vi "Quiz.vi"() -> ()   [LabVIEW 2020]
uses:
  <vilib>/Utility/error.llb/whitespace.ctl
panel:
  in  "array 3":string[](array[string])
  in  "array 2":string[](array[string])
  in  "array":string[](array[string])
  out "x+y":i16
  in  "Boolean 6":bool
  in  "Boolean 5":bool
  in  "Boolean 4":bool
  out "Boolean 3":bool
  out "Boolean 2":bool
  out "Boolean":bool
  out "Array 2":string[](array[string])
  out "number":dbl
  out "Numeric":i32
  in  "?":string
  in  "?":bool
  out "?":string
  in  "?":string
  # "Ingresar trama"
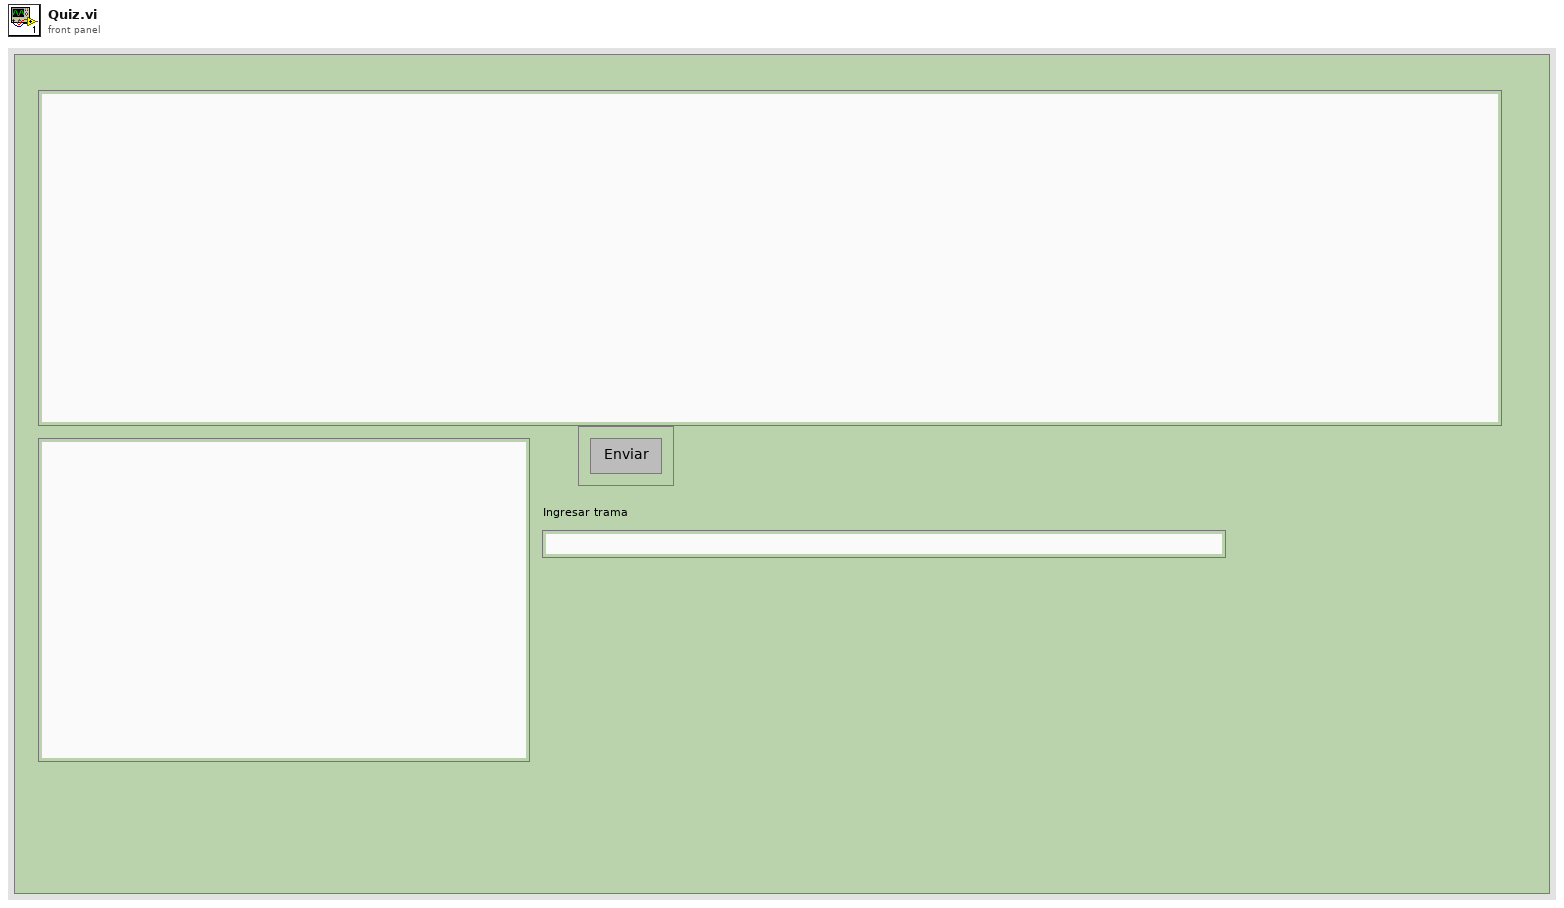
[diagram p1: front panel]
types:
  T1 = enum8{"Enabled", "Disabled", "Disabled and Grayed Out"}
  T2 = typedef "whitespace.ctl" = u16
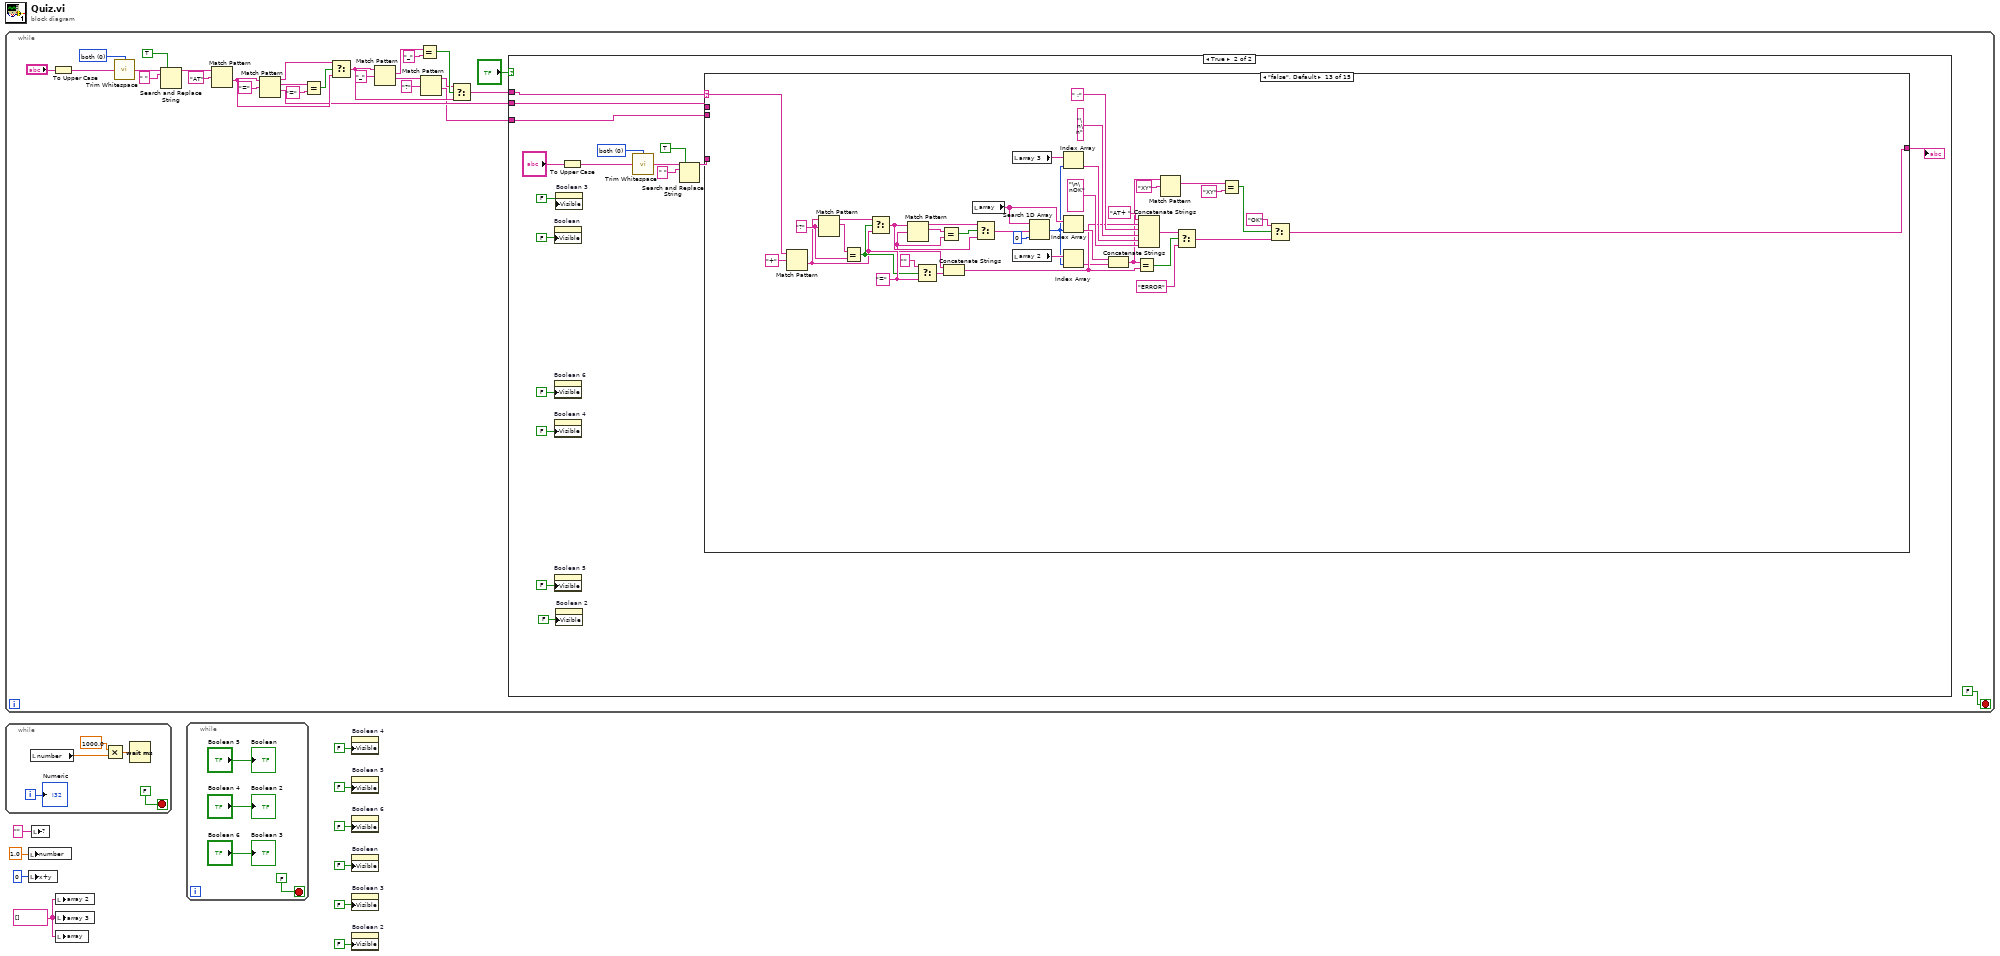
[diagram p0: block diagram]
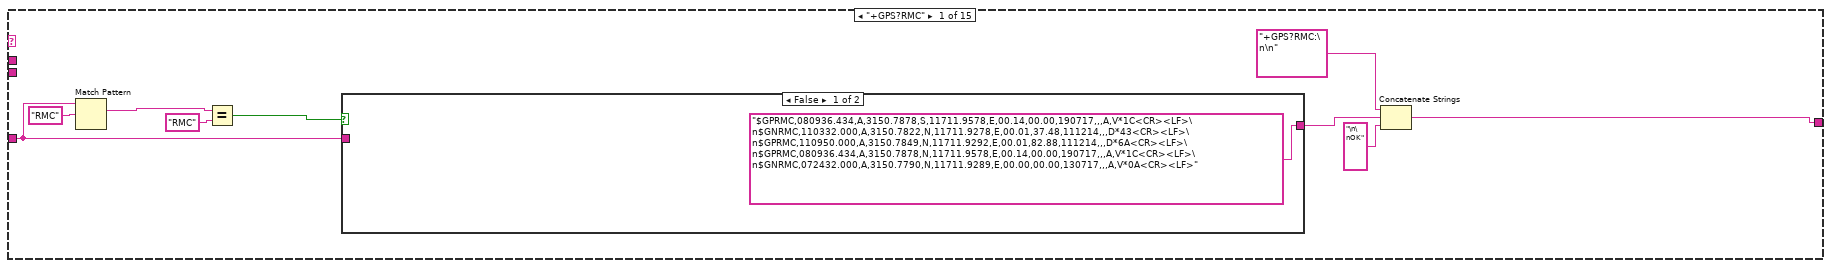
[diagram p3: hidden frame]
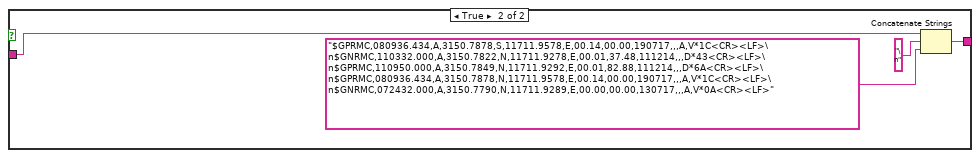
[diagram p4: hidden frame]
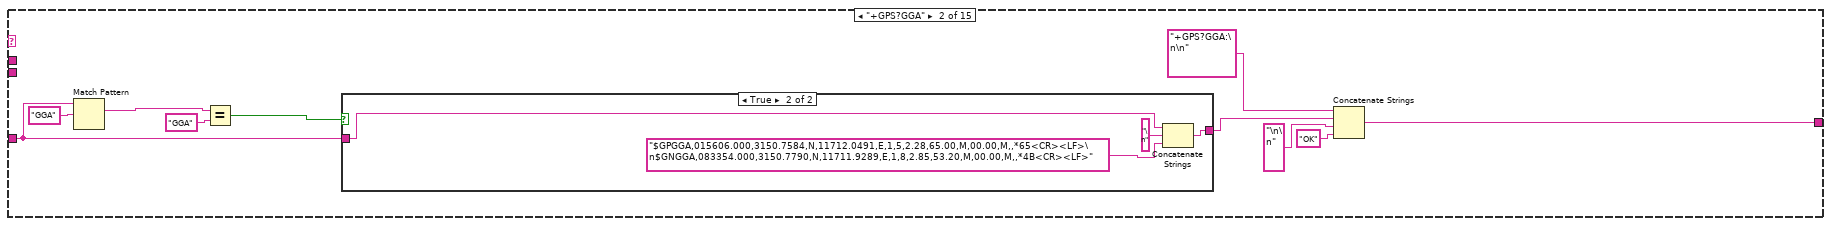
[diagram p5: hidden frame]
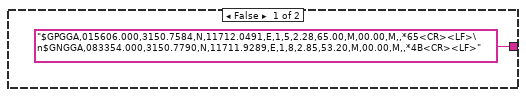
[diagram p6: hidden frame]
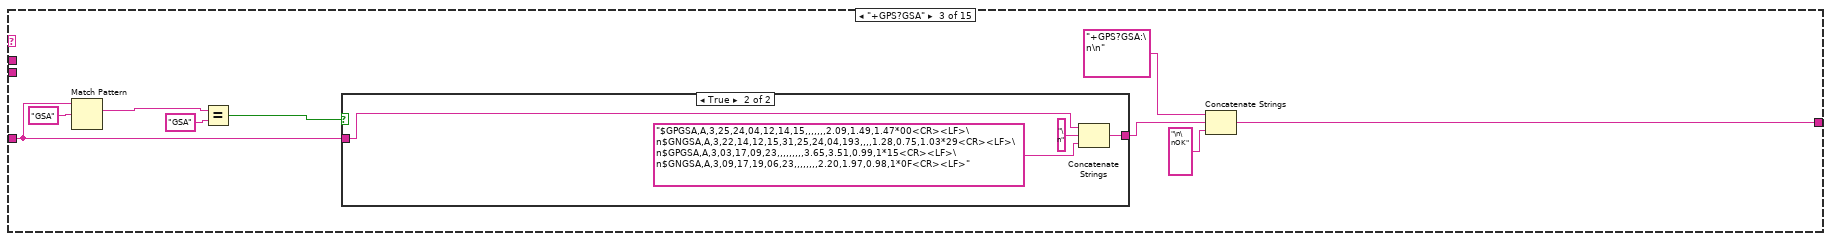
[diagram p7: hidden frame]
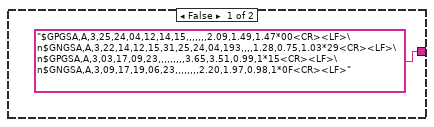
[diagram p8: hidden frame]
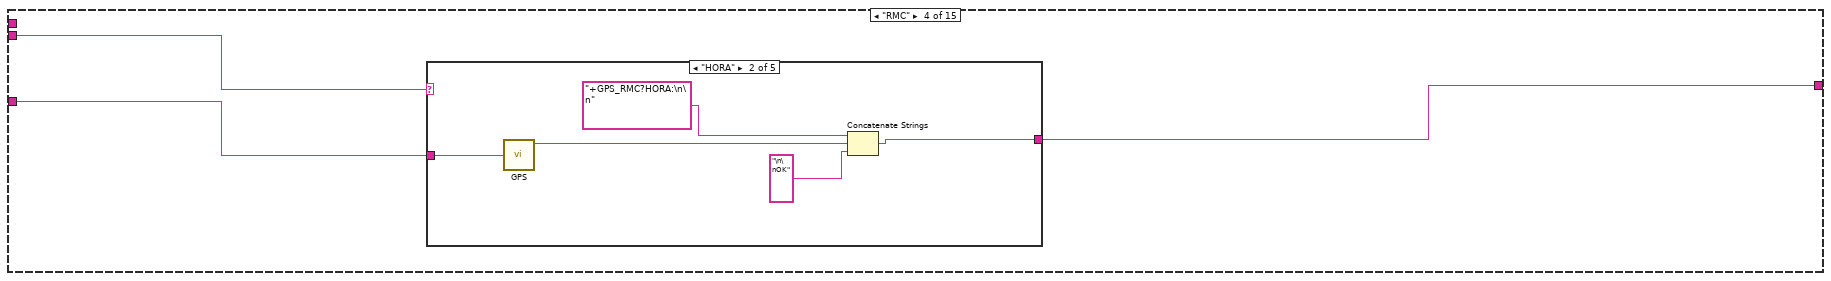
[diagram p9: hidden frame]
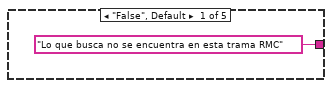
[diagram p10: hidden frame]
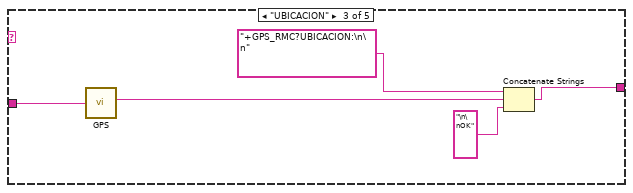
[diagram p11: hidden frame]
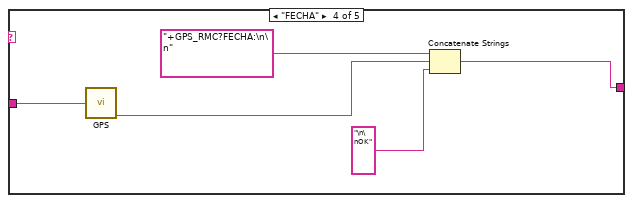
[diagram p12: hidden frame]
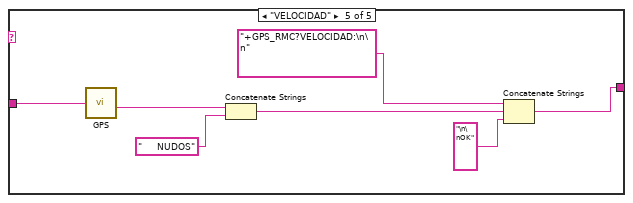
[diagram p13: hidden frame]
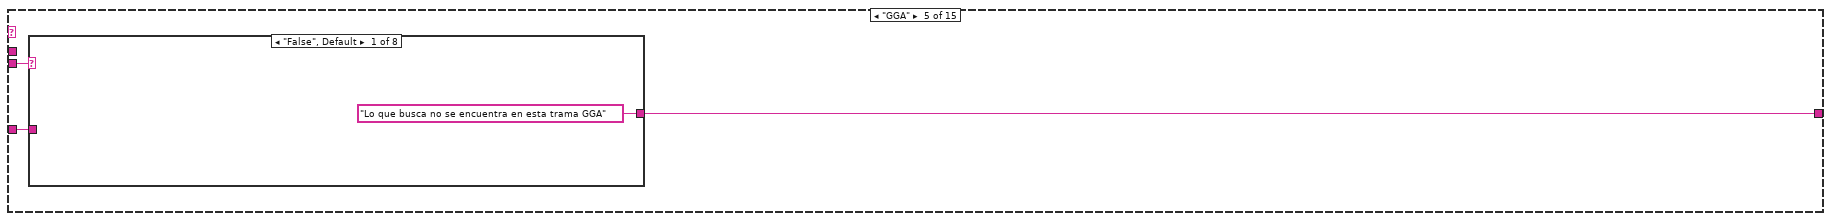
[diagram p14: hidden frame]
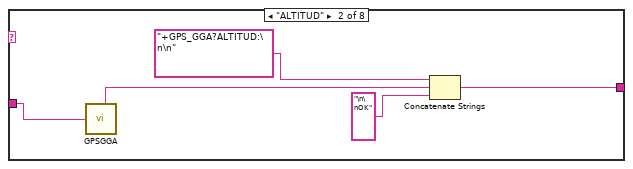
[diagram p15: hidden frame]
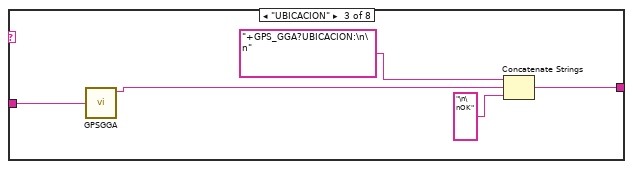
[diagram p16: hidden frame]
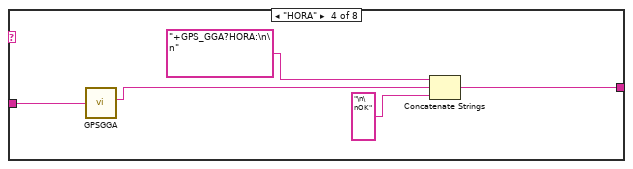
[diagram p17: hidden frame]
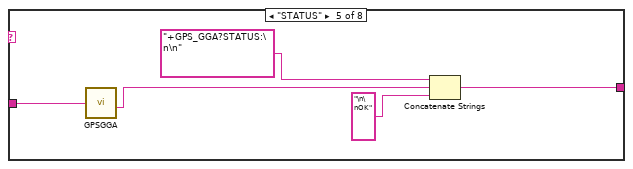
[diagram p18: hidden frame]
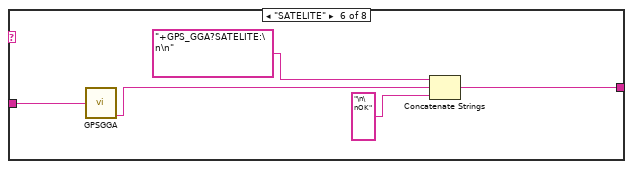
[diagram p19: hidden frame]
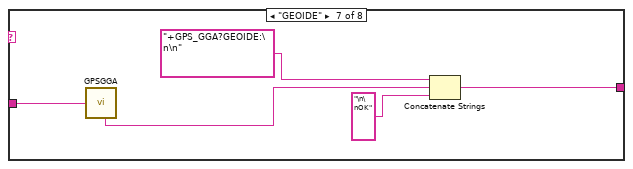
[diagram p20: hidden frame]
diagram:
  w1 = string[] [] ("Array")
  n1 = while {
    stop <- FALSE stop-if-true
    w17 = T2 0 items=["both", "start of string", "end of string"] ("location (both)")
    n2 = To Upper Case(1:"?") -> (0:w13:string)
    n3 = call <vilib>:"Trim Whitespace.vi"("string"=w13, "location (both)"=w17) -> ("trimmed string"=w16:string)
    n4 = Search and Replace String(replace all?=TRUE ("replace all? (F)"), input string=w16, search string=" ") -> (result string=w12:string)  [unwired: 5 in, 3 out]
    n5 = Match Pattern(string=w12, regular expression="AT" ("string")) -> (after substring=w28:string)  [unwired: 1 in, 3 out]
    n6 = Match Pattern(string=w28, regular expression="=") -> (before substring=w29:string, match substring=w32:string, after substring=w27:string)  [unwired: 1 in, 1 out]
    n7 = Equal?(x=w32, y="=") -> (x = y?=w30:bool)
    n8 = Select(t=w29, s=w30, f=w28) -> (s? t:f=w22:string)
    n9 = Match Pattern(string=w22, regular expression="_") -> (match substring=w25:string, after substring=w21:string)  [unwired: 1 in, 2 out]
    n10 = Equal?(x=w25, y="_") -> (x = y?=w23:bool)
    n11 = Match Pattern(string=w21, regular expression="?") -> (before substring=w19:string, after substring=w18:string)  [unwired: 1 in, 2 out]
    n12 = Select(t=w19, s=w23, f=w22) -> (s? t:f=w11:string)
    n13 = case shown="True" "?" {
      tunnel: w11 -> [_ w54]
      tunnel: w27 -> [_ w53]
      tunnel: w18 -> [_ w51]
      frame False {
      }
      frame True {
        w46 = T2 0 items=["both", "start of string", "end of string"] ("location (both)")
        n14 = property on="Boolean" class="Bool (strict)"("Visible"=FALSE) -> ()  [unwired: 2 in, 2 out]
        n15 = property on="Boolean 6" class="Bool (strict)"("Visible"=FALSE) -> ()  [unwired: 2 in, 2 out]
        n16 = property on="Boolean 4" class="Bool (strict)"("Visible"=FALSE) -> ()  [unwired: 2 in, 2 out]
        n17 = property on="Boolean 5" class="Bool (strict)"("Visible"=FALSE) -> ()  [unwired: 2 in, 2 out]
        n18 = property on="Boolean 3" class="Bool (strict)"("Visible"=FALSE) -> ()  [unwired: 2 in, 2 out]
        n19 = property on="Boolean 2" class="Bool (strict)"("Visible"=FALSE) -> ()  [unwired: 2 in, 2 out]
        n20 = To Upper Case(1:"?") -> (0:w50:string)
        n21 = call <vilib>:"Trim Whitespace.vi"("string"=w50, "location (both)"=w46) -> ("trimmed string"=w47:string)
        n22 = Search and Replace String(replace all?=TRUE ("replace all? (F)"), input string=w47, search string=" ") -> (result string=w45:string)  [unwired: 5 in, 3 out]
        n23 = case shown="\"false\", Default" w54 {
          selector: w54 -> [_ _ _ _ _ _ _ _ _ _ _ _ w378 _ _]
          tunnel: [w56 w71 w85 w98 w124 w164 w255 w262 w274 "" "" w318 w340 w379 "AT:\n\nOk"] -> w52
          tunnel: w45 -> [w61 w74 w88 w100 w126 w162 _ _ _ _ _ _ _ _ _]
          tunnel: w53 -> [_ _ _ _ _ _ _ w268 _ _ _ w316 _ _ _]
          tunnel: w51 -> [_ _ _ w99 w125 w165 _ _ _ _ _ _ _ _ _]
          frame "+GPS?RMC" {
            n24 = Match Pattern(string=w61, regular expression="RMC") -> (match substring=w59:string)  [unwired: 1 in, 3 out]
            n25 = Equal?(x=w59, y="RMC") -> (x = y?=w62:bool)
            n26 = case shown="False" w62 {
              tunnel: w61 -> [_ w66]
              tunnel: ["$GPRMC,080936.434,A,3150.7878,S,11711.9578,E,00.14,00.00,190717,,,A,V*1C<CR><LF>\n$GNRMC,110332.000,A,3150.7822,N,11711.9278,E,00.01,37.48,111214,,,D*43<CR><LF>\n$GPRMC,110950.000,A,3150.7849,N,11711.9292,E,00.01,82.88,111214,,,D*6A<CR><LF>\n$GPRMC,080936.434,A,3150.7878,N,11711.9578,E,00.14,00.00,190717,,,A,V*1C<CR><LF>\n$GNRMC,072432.000,A,3150.7790,N,11711.9289,E,00.00,00.00,130717,,,A,V*0A<CR><LF>" w68] -> w57
              frame False {
              }
              frame True {
                n27 = Concatenate Strings(w66, "\n" ("string"), "$GPRMC,080936.434,A,3150.7878,S,11711.9578,E,00.14,00.00,190717,,,A,V*1C<CR><LF>\n$GNRMC,110332.000,A,3150.7822,N,11711.9278,E,00.01,37.48,111214,,,D*43<CR><LF>\n$GPRMC,110950.000,A,3150.7849,N,11711.9292,E,00.01,82.88,111214,,,D*6A<CR><LF>\n$GPRMC,080936.434,A,3150.7878,N,11711.9578,E,00.14,00.00,190717,,,A,V*1C<CR><LF>\n$GNRMC,072432.000,A,3150.7790,N,11711.9289,E,00.00,00.00,130717,,,A,V*0A<CR><LF>") -> (w68:string)
              }
            }
            n28 = Concatenate Strings("+GPS?RMC:\n\n" ("string"), w57, "\n\nOK" ("string")) -> (w56:string)
          }
          frame "+GPS?GGA" {
            n29 = Match Pattern(string=w74, regular expression="GGA") -> (match substring=w75:string)  [unwired: 1 in, 3 out]
            n30 = Equal?(x=w75, y="GGA") -> (x = y?=w76:bool)
            n31 = case shown="True" w76 {
              tunnel: w74 -> [_ w81]
              tunnel: ["$GPGGA,015606.000,3150.7584,N,11712.0491,E,1,5,2.28,65.00,M,00.00,M,,*65<CR><LF>\n$GNGGA,083354.000,3150.7790,N,11711.9289,E,1,8,2.85,53.20,M,00.00,M,,*4B<CR><LF>" w83] -> w72
              frame False {
              }
              frame True {
                n32 = Concatenate Strings(w81, "\n" ("string"), "$GPGGA,015606.000,3150.7584,N,11712.0491,E,1,5,2.28,65.00,M,00.00,M,,*65<CR><LF>\n$GNGGA,083354.000,3150.7790,N,11711.9289,E,1,8,2.85,53.20,M,00.00,M,,*4B<CR><LF>") -> (w83:string)
              }
            }
            n33 = Concatenate Strings("+GPS?GGA:\n\n" ("string"), w72, "\n\n" ("string"), "OK" ("string")) -> (w71:string)
          }
          frame "+GPS?GSA" {
            n34 = Match Pattern(string=w88, regular expression="GSA") -> (match substring=w89:string)  [unwired: 1 in, 3 out]
            n35 = Equal?(x=w89, y="GSA") -> (x = y?=w90:bool)
            n36 = case shown="True" w90 {
              tunnel: w88 -> [_ w95]
              tunnel: ["$GPGSA,A,3,25,24,04,12,14,15,,,,,,,2.09,1.49,1.47*00<CR><LF>\n$GNGSA,A,3,22,14,12,15,31,25,24,04,193,,,,1.28,0.75,1.03*29<CR><LF>\n$GPGSA,A,3,03,17,09,23,,,,,,,,,3.65,3.51,0.99,1*15<CR><LF>\n$GNGSA,A,3,09,17,19,06,23,,,,,,,,2.20,1.97,0.98,1*0F<CR><LF>" w96] -> w86
              frame False {
              }
              frame True {
                n37 = Concatenate Strings(w95, "\n" ("string"), "$GPGSA,A,3,25,24,04,12,14,15,,,,,,,2.09,1.49,1.47*00<CR><LF>\n$GNGSA,A,3,22,14,12,15,31,25,24,04,193,,,,1.28,0.75,1.03*29<CR><LF>\n$GPGSA,A,3,03,17,09,23,,,,,,,,,3.65,3.51,0.99,1*15<CR><LF>\n$GNGSA,A,3,09,17,19,06,23,,,,,,,,2.20,1.97,0.98,1*0F<CR><LF>") -> (w96:string)
              }
            }
            n38 = Concatenate Strings("+GPS?GSA:\n\n" ("string"), w86, "\n\nOK" ("string")) -> (w85:string)
          }
          frame "RMC" {
            n39 = case shown="\"HORA\"" w99 {
              tunnel: w100 -> [_ w106 w111 w116 w123]
              tunnel: ["Lo que busca no se encuentra en esta trama RMC" w102 w107 w112 w117] -> w98
              frame "False", Default {
              }
              frame "HORA" {
                n40 = call "GPS.vi"("String"=w106) -> ("Hora"=w103:string)  [unwired: 3 out]
                n41 = Concatenate Strings("+GPS_RMC?HORA:\n\n" ("string"), w103, "\n\nOK" ("string")) -> (w102:string)
              }
              frame "UBICACION" {
                n42 = call "GPS.vi"("String"=w111) -> ("Ubicación"=w108:string)  [unwired: 3 out]
                n43 = Concatenate Strings("+GPS_RMC?UBICACION:\n\n" ("string"), w108, "\n\nOK" ("string")) -> (w107:string)
              }
              frame "FECHA" {
                n44 = call "GPS.vi"("String"=w116) -> ("Fecha"=w113:string)  [unwired: 3 out]
                n45 = Concatenate Strings("+GPS_RMC?FECHA:\n\n" ("string"), w113, "\n\nOK" ("string")) -> (w112:string)
              }
              frame "VELOCIDAD" {
                n46 = call "GPS.vi"("String"=w123) -> ("Velocidad"=w121:string)  [unwired: 3 out]
                n47 = Concatenate Strings(w121, "     NUDOS" ("string")) -> (w118:string)
                n48 = Concatenate Strings("+GPS_RMC?VELOCIDAD:\n\n" ("string"), w118, "\n\nOK" ("string")) -> (w117:string)
              }
            }
          }
          frame "GGA" {
            n49 = case shown="\"False\", Default" w125 {
              tunnel: w126 -> [_ w132 w137 w142 w147 w152 w157 _]
              tunnel: ["Lo que busca no se encuentra en esta trama GGA" w129 w133 w138 w143 w148 w154 w158] -> w124
              frame "False", Default {
              }
              frame "ALTITUD" {
                n50 = call "GPSGGA.vi"("String"=w132) -> ("Altitud"=w128:string)  [unwired: 5 out]
                n51 = Concatenate Strings("+GPS_GGA?ALTITUD:\n\n" ("string"), w128, "\n\nOK" ("string")) -> (w129:string)
              }
              frame "UBICACION" {
                n52 = call "GPSGGA.vi"("String"=w137) -> ("Ubicación"=w134:string)  [unwired: 5 out]
                n53 = Concatenate Strings("+GPS_GGA?UBICACION:\n\n" ("string"), w134, "\n\nOK" ("string")) -> (w133:string)
              }
              frame "HORA" {
                n54 = call "GPSGGA.vi"("String"=w142) -> ("Hora"=w139:string)  [unwired: 5 out]
                n55 = Concatenate Strings("+GPS_GGA?HORA:\n\n" ("string"), w139, "\n\nOK" ("string")) -> (w138:string)
              }
              frame "STATUS" {
                n56 = call "GPSGGA.vi"("String"=w147) -> ("Fix Status"=w144:string)  [unwired: 5 out]
                n57 = Concatenate Strings("+GPS_GGA?STATUS:\n\n" ("string"), w144, "\n\nOK" ("string")) -> (w143:string)
              }
              frame "SATELITE" {
                n58 = call "GPSGGA.vi"("String"=w152) -> ("# Satelite"=w149:string)  [unwired: 5 out]
                n59 = Concatenate Strings("+GPS_GGA?SATELITE:\n\n" ("string"), w149, "\n\nOK" ("string")) -> (w148:string)
              }
              frame "GEOIDE" {
                n60 = call "GPSGGA.vi"("String"=w157) -> ("Sep Geoide"=w153:string)  [unwired: 5 out]
                n61 = Concatenate Strings("+GPS_GGA?GEOIDE:\n\n" ("string"), w153, "\n\nOK" ("string")) -> (w154:string)
              }
              frame "VELOCIDAD" {
                n62 = Concatenate Strings("+GPS_GGA?VELOCIDAD:\n\n" ("string"), "La trama GGA no tiene velocidad", "\n\nOK" ("string")) -> (w158:string)
              }
            }
          }
          frame "GSA" {
            n63 = call "GPSGSA.vi"("string"=w162) -> ("Array"=→"Array 2":string[])
            n64 = case shown="\"SATELITE1\"" w165 {
              tunnel: ["Lo que busca no se encuentra en la trama GSA" w167 w173 w180 w185 w192 w198 w204 w210 w216 w222 w228 w234 w240 w245 w250] -> w164
              frame "False", Default {
              }
              frame "MODO" {
                n65 = local read "Array 2"() -> (w172:string[])
                n66 = Index Array(array=w172, index=0) -> (element=w168:string)
                n67 = Concatenate Strings("+GPS_GSA?MODO:\n\n" ("string"), w168, "\n\nOK" ("string")) -> (w167:string)
              }
              frame "STATUS" {
                n68 = local read "Array 2"() -> (w178:string[])
                n69 = Index Array(array=w178, index=1) -> (element=w174:string)
                n70 = Concatenate Strings("+GPS_GSA?STATUS:\n\n" ("string"), w174, "\n\nOK" ("string")) -> (w173:string)
              }
              frame "SATELITE1" {
                n71 = local read "Array 2"() -> (w184:string[])
                n72 = Index Array(array=w184, index=2) -> (element=w179:string)
                n73 = Concatenate Strings("+GPS_GSA?SATELITE1:\n\n" ("string"), w179, "\n\nOK" ("string")) -> (w180:string)
              }
              frame "SATELITE2" {
                n74 = local read "Array 2"() -> (w190:string[])
                n75 = Index Array(array=w190, index=3) -> (element=w186:string)
                n76 = Concatenate Strings("+GPS_GSA?SATELITE2:\n\n" ("string"), w186, "\n\nOK" ("string")) -> (w185:string)
              }
              frame "SATELITE3" {
                n77 = local read "Array 2"() -> (w196:string[])
                n78 = Index Array(array=w196, index=4) -> (element=w191:string)
                n79 = Concatenate Strings("+GPS_GSA?SATELITE3:\n\n" ("string"), w191, "\n\nOK" ("string")) -> (w192:string)
              }
              frame "SATELITE4" {
                n80 = local read "Array 2"() -> (w202:string[])
                n81 = Index Array(array=w202, index=5) -> (element=w197:string)
                n82 = Concatenate Strings("+GPS_GSA?SATELITE4:\n\n" ("string"), w197, "\n\nOK" ("string")) -> (w198:string)
              }
              frame "SATELITE5" {
                n83 = local read "Array 2"() -> (w208:string[])
                n84 = Index Array(array=w208, index=6) -> (element=w203:string)
                n85 = Concatenate Strings("+GPS_GSA?SATELITE5:\n\n" ("string"), w203, "\n\nOK" ("string")) -> (w204:string)
              }
              frame "SATELITE6" {
                n86 = local read "Array 2"() -> (w214:string[])
                n87 = Index Array(array=w214, index=7) -> (element=w209:string)
                n88 = Concatenate Strings("+GPS_GSA?SATELITE6:\n\n" ("string"), w209, "\n\nOK" ("string")) -> (w210:string)
              }
              frame "SATELITE7" {
                n89 = local read "Array 2"() -> (w220:string[])
                n90 = Index Array(array=w220, index=8) -> (element=w215:string)
                n91 = Concatenate Strings("+GPS_GSA?SATELITE7:\n\n" ("string"), w215, "\n\nOK" ("string")) -> (w216:string)
              }
              frame "SATELITE8" {
                n92 = local read "Array 2"() -> (w226:string[])
                n93 = Index Array(array=w226, index=9) -> (element=w221:string)
                n94 = Concatenate Strings("+GPS_GSA?SATELITE8:\n\n" ("string"), w221, "\n\nOK" ("string")) -> (w222:string)
              }
              frame "SATELITE9" {
                n95 = local read "Array 2"() -> (w232:string[])
                n96 = Index Array(array=w232, index=10) -> (element=w227:string)
                n97 = Concatenate Strings("+GPS_GSA?SATELITE9:\n\n" ("string"), w227, "\n\nOK" ("string")) -> (w228:string)
              }
              frame "SATELITE10" {
                n98 = local read "Array 2"() -> (w238:string[])
                n99 = Index Array(array=w238, index=11) -> (element=w233:string)
                n100 = Concatenate Strings("+GPS_GSA?SATELITE10:\n\n" ("string"), w233, "\n\nOK" ("string")) -> (w234:string)
              }
              frame "SATELITE11" {
                n101 = local read "Array 2"() -> (w244:string[])
                n102 = Index Array(array=w244, index=12) -> (element=w239:string)
                n103 = Concatenate Strings("+GPS_GSA?SATELITE11:\n\n" ("string"), w239, "\n\nOK" ("string")) -> (w240:string)
              }
              frame "VELOCIDAD" {
                n104 = Concatenate Strings("+GPS_GSA?VELOCIDAD:\n\n" ("string"), "La trama GSA no tiene velocidad", "\n\nOK" ("string")) -> (w245:string)
              }
              frame "SATELITE12" {
                n105 = local read "Array 2"() -> (w254:string[])
                n106 = Index Array(array=w254, index=13) -> (element=w249:string)
                n107 = Concatenate Strings("+GPS_GSA?SATELITE12:\n\n" ("string"), w249, "\n\nOK" ("string")) -> (w250:string)
              }
            }
          }
          frame "+TIMER" {
            n108 = Format Date/Time String() -> (date/time string=w258:string)  [unwired: 3 in]
            n109 = Concatenate Strings(w258, "\n\n" ("string"), "OK" ("string")) -> (w256:string)
            n110 = Concatenate Strings("+TIMER:\n\n" ("string"), w256) -> (w255:string)
          }
          frame "+CONT" {
            n111 = Fract/Exp String To Number(string=w268, default (0 dbl)=1.0 ("default (0 DBL)")) -> (number=w265:dbl)  [unwired: 2 in, 1 out]
            "number" <- w265
            n112 = Number To Decimal String(number=w265) -> (decimal integer string=w264:string)  [unwired: 1 in]
            n113 = Concatenate Strings("+CONT:\n\nEl contador aumenta cada ", w264, "   seg" ("string"), "\n\nOK" ("string")) -> (w262:string)
          }
          frame "+CONT?" {
            n114 = local read "Numeric"() -> (w276:i32)
            n115 = Number To Decimal String(number=w276) -> (decimal integer string=w273:string)  [unwired: 1 in]
            n116 = Concatenate Strings("El valor actual del contador es:" ("string"), w273, "  seg" ("string")) -> (w270:string)
            n117 = Concatenate Strings("+CONT?:\n\n" ("string"), w270, "\n\nOK" ("string")) -> (w274:string)
          }
          frame "+ESTADO?" {
            n118 = property on="Boolean 2" class="Bool (strict)"("Visible"=TRUE) -> ()  [unwired: 2 in, 2 out]
            n119 = property on="Boolean 3" class="Bool (strict)"("Visible"=TRUE) -> ()  [unwired: 2 in, 2 out]
            n120 = property on="Boolean" class="Bool (strict)"("Visible"=TRUE) -> ()  [unwired: 2 in, 2 out]
            n121 = property on="Boolean 6" class="Bool (strict)"("Visible"=TRUE) -> ()  [unwired: 2 in, 2 out]
            n122 = property on="Boolean 4" class="Bool (strict)"("Visible"=TRUE) -> ()  [unwired: 2 in, 2 out]
            n123 = property on="Boolean 5" class="Bool (strict)"("Visible"=TRUE) -> ()  [unwired: 2 in, 2 out]
            n124 = property on="Boolean 3" class="Bool (strict)"("DisabledEnum"=T1."Disabled" ("Disabled")) -> ()  [unwired: 2 in, 2 out]
            n125 = property on="Boolean 6" class="Bool (strict)"("DisabledEnum"=T1."Disabled" ("Disabled")) -> ()  [unwired: 2 in, 2 out]
            n126 = property on="Boolean 2" class="Bool (strict)"("DisabledEnum"=T1."Disabled" ("Disabled")) -> ()  [unwired: 2 in, 2 out]
            n127 = property on="Boolean 4" class="Bool (strict)"("DisabledEnum"=T1."Disabled" ("Disabled")) -> ()  [unwired: 2 in, 2 out]
            n128 = property on="Boolean" class="Bool (strict)"("DisabledEnum"=T1."Disabled" ("Disabled")) -> ()  [unwired: 2 in, 2 out]
            n129 = property on="Boolean 5" class="Bool (strict)"("DisabledEnum"=T1."Disabled" ("Disabled")) -> ()  [unwired: 2 in, 2 out]
          }
          frame "+CAMBIAR" {
            n130 = property on="Boolean 2" class="Bool (strict)"("Visible"=TRUE) -> ()  [unwired: 2 in, 2 out]
            n131 = property on="Boolean 3" class="Bool (strict)"("Visible"=TRUE) -> ()  [unwired: 2 in, 2 out]
            n132 = property on="Boolean" class="Bool (strict)"("Visible"=TRUE) -> ()  [unwired: 2 in, 2 out]
            n133 = property on="Boolean 6" class="Bool (strict)"("Visible"=TRUE) -> ()  [unwired: 2 in, 2 out]
            n134 = property on="Boolean 4" class="Bool (strict)"("Visible"=TRUE) -> ()  [unwired: 2 in, 2 out]
            n135 = property on="Boolean 5" class="Bool (strict)"("Visible"=TRUE) -> ()  [unwired: 2 in, 2 out]
            n136 = property on="Boolean 3" class="Bool (strict)"("DisabledEnum"=T1."Enabled" ("Disabled")) -> ()  [unwired: 2 in, 2 out]
            n137 = property on="Boolean 6" class="Bool (strict)"("DisabledEnum"=T1."Enabled" ("Disabled")) -> ()  [unwired: 2 in, 2 out]
            n138 = property on="Boolean 2" class="Bool (strict)"("DisabledEnum"=T1."Enabled" ("Disabled")) -> ()  [unwired: 2 in, 2 out]
            n139 = property on="Boolean 4" class="Bool (strict)"("DisabledEnum"=T1."Enabled" ("Disabled")) -> ()  [unwired: 2 in, 2 out]
            n140 = property on="Boolean" class="Bool (strict)"("DisabledEnum"=T1."Enabled" ("Disabled")) -> ()  [unwired: 2 in, 2 out]
            n141 = property on="Boolean 5" class="Bool (strict)"("DisabledEnum"=T1."Enabled" ("Disabled")) -> ()  [unwired: 2 in, 2 out]
          }
          frame "+GUARDAR" {
            w311 = "OK" ("y")
            n142 = flat-sequence {
              tunnel: [w322] -> w317
              tunnel: w317 -> [w331]
              tunnel: w316 -> [w333]
              tunnel: [w328] -> w315
              tunnel: [w324] -> w314
              tunnel: [w324] -> w313
              tunnel: [w323] -> w305
              frame #0 {
                n143 = local read "x+y"() -> (w322:i16)
              }
              frame #1 {
                n144 = Match Pattern(string=w333, regular expression=",") -> (before substring=w328:string, after substring=w335:string)  [unwired: 1 in, 2 out]
                n145 = Insert Into Array(array="array", index=w331, new element=w328) -> (w329:string[])
                n146 = Match Pattern(string=w335, regular expression=",") -> (before substring=w323:string, after substring=w324:string)  [unwired: 1 in, 2 out]
                n147 = property on="array" class="Arr (strict)"("Value"=w329) -> ()  [unwired: 2 in, 2 out]
                n148 = Insert Into Array(array="array 2", index=w331, new element=w323) -> (w330:string[])
                n149 = Insert Into Array(array="array 3", index=w331, new element=w324) -> (w325:string[])
                n150 = property on="array 2" class="Arr (strict)"("Value"=w330) -> ()  [unwired: 2 in, 2 out]
                n151 = property on="array 3" class="Arr (strict)"("Value"=w325) -> ()  [unwired: 2 in, 2 out]
              }
              frame #2 {
                n152 = local read "x+y"() -> (w338:i16)
                n153 = Add(x=w338, y=i16 1) -> (x+y=→"x+y":i16)
              }
            }
            n154 = Equal?(x=w305, y="XY") -> (x = y?=w306:bool)
            n155 = Select(t="=X, Y", s=w306, f=w305) -> (s? t:f=w303:string)
            n156 = Equal?(x=w313, y=w311) -> (x = y?=w312:bool)
            n157 = Select(t="", s=w312, f=w311) -> (s? t:f=w308:string)
            n158 = Concatenate Strings("AT+" ("string"), w315, w303, "\n\n\n", w314, "\n", "\n" ("string"), w308) -> (w318:string)
          }
          frame "false", Default {
            w356 = "=" ("regular expression")
            w371 = "?" ("regular expression")
            n159 = Match Pattern(string=w378, regular expression="+") -> (after substring=w350:string)  [unwired: 1 in, 3 out]
            n160 = Match Pattern(string=w350, regular expression=w371) -> (before substring=w375:string, match substring=w376:string)  [unwired: 1 in, 2 out]
            n161 = Equal?(x=w376, y=w371) -> (x = y?=w354:bool)
            n162 = Select(t=w375, s=w354, f=w350) -> (s? t:f=w372:string)
            n163 = Match Pattern(string=w372, regular expression=w356) -> (before substring=w373:string, match substring=w374:string)  [unwired: 1 in, 2 out]
            n164 = Select(t="", s=w354, f=w356) -> (s? t:f=w351:string)
            n165 = Equal?(x=w374, y=w356) -> (x = y?=w357:bool)
            n166 = Concatenate Strings(w350, w351) -> (w349:string)
            n167 = local read "array"() -> (w368:string[])
            n168 = Select(t=w373, s=w357, f=w372) -> (s? t:f=w370:string)
            n169 = local read "array 3"() -> (w366:string[])
            n170 = local read "array 2"() -> (w367:string[])
            n171 = Search 1D Array(1D array=w368, element=w370, start index (0)=0) -> (index of element=w365:i32)
            n172 = Index Array(array=w366, index=w365) -> (element=w360:string)
            n173 = Index Array(array=w368, index=w365) -> (element=w352:string)
            n174 = Index Array(array=w367, index=w365) -> (element=w348:string)
            n175 = Concatenate Strings(w352, w348) -> (w346:string)
            n176 = Equal?(x=w346, y=w349) -> (x = y?=w364:bool)
            n177 = Concatenate Strings("AT+ " ("string"), w349, " :" ("string"), "\n\n" ("string"), w360, "\n\nOK" ("string")) -> (w359:string)
            n178 = Match Pattern(string=w346, regular expression="XY") -> (match substring=w344:string)  [unwired: 1 in, 3 out]
            n179 = Select(t=w359, s=w364, f="ERROR") -> (s? t:f=w342:string)
            n180 = Equal?(x=w344, y="XY") -> (x = y?=w343:bool)
            n181 = Select(t="OK", s=w343, f=w342) -> (s? t:f=w340:string)
          }
          frame "+HELP" {
            n182 = Concatenate Strings("+HELP:\n\nCOMANDO                                                              DESCRIPCIÓN\n      AT                                                                               OK\nAT +GPS?RMC                     |     Consulta la trama RMC completa \nAT +GPS?GGA                     |     Consulta la trama GGA completa  \nAT +GPS?GSA                      |     Consulta la trama GSA completa \nAT +GPS_RMC?X                 |     Consulta el campo X en la trama RMC (X= hora, fecha, velocidad, ubicacion) \nAT +GPS_GGA?X                  |     Consulta el campo X en la trama GGA(X= hora, altitud, ubicacion, velocidad, status, satelite, fecha) \nAT +GPS_GSA?X                  |     Consulta el campo X en la trama GSA (X= modo, status ,satelite1,satelite2, satelite3, satelite4, satelite5, satelite6, satelite7, satelite8, satelite9, satelite10, satelite11, satelite12)\nAT +TIMER                              |     Consulta la hora y fecha del sistema \nAT +CONT=X                          |     Modifica el tiempo de incremento del contador en X tiempo \nAT +CONT?                             |     Lee  la variable del contador \nAT +ESTADO?                        |     Lee el estado de los leds y los pulsadores\nAT +CAMBIAR                         |     Modifica el estado de los leds y los pulsadores \nAT +GUARDAR=X , Y, Z         |     Guarda el comando que ingrese el usuario(X=Nombre del comando, Y=Tipo de comando, Z=Respuesta del comando)", "\n\n" ("string"), "OK" ("string")) -> (w379:string)
          }
          frame "" {
          }
        }
        "?" <- w52
      }
    }
  }
  n183 = while {
    i -> [w385]
    stop <- FALSE stop-if-true
    n184 = local read "number"() -> (w388:dbl)
    n185 = Multiply(x=1000.0, y=w388) -> (x*y=w387:dbl)
    n186 = Wait (ms)(milliseconds to wait=w387) -> ()  [unwired: 1 out]
    "Numeric" <- w385
  }
  n187 = local write "number"(1.0 ("number")) -> ()
  n188 = local write "x+y"(i16 0 ("x+y")) -> ()
  n189 = local write item#1("" ("String 2")) -> ()
  n190 = local write "array 2"(w1) -> ()
  n191 = local write "array 3"(w1) -> ()
  n192 = local write "array"(w1) -> ()
  n193 = while {
    stop <- FALSE stop-if-true
    "Boolean" <- "Boolean 5"
    "Boolean 2" <- "Boolean 4"
    "Boolean 3" <- "Boolean 6"
  }
  n194 = property on="Boolean 4" class="Bool (strict)"("Visible"=FALSE) -> ()  [unwired: 2 in, 2 out]
  n195 = property on="Boolean 5" class="Bool (strict)"("Visible"=FALSE) -> ()  [unwired: 2 in, 2 out]
  n196 = property on="Boolean 6" class="Bool (strict)"("Visible"=FALSE) -> ()  [unwired: 2 in, 2 out]
  n197 = property on="Boolean" class="Bool (strict)"("Visible"=FALSE) -> ()  [unwired: 2 in, 2 out]
  n198 = property on="Boolean 3" class="Bool (strict)"("Visible"=FALSE) -> ()  [unwired: 2 in, 2 out]
  n199 = property on="Boolean 2" class="Bool (strict)"("Visible"=FALSE) -> ()  [unwired: 2 in, 2 out]
